vi "read data type.vi"(8 "error in":errorcluster, 11 "system tag in":refnum<class "tag descriptor.lvclass">) -> (0 "error out":errorcluster, 2 "data type":T1, 3 "system tag out":refnum<class "tag descriptor.lvclass">)   [LabVIEW 2013, in "tag bus.lvlib" / "tag descriptor.lvclass"]
doc: "Read the value of the data type enum in a given tag descriptor."
uses:
  tag descriptor.lvclass
  Data Type.ctl
  tag descriptor.lvclass/tag descriptor.ctl
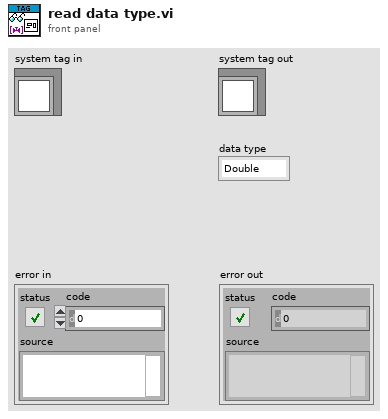
[diagram p1: front panel]
types:
  T1 = typedef "tag bus.lvlib/tag descriptor.lvclass/Data Type.ctl" = enum16{"Double", "Single", "I64", "I32", "I16", "I8", "U64", "U32", "U16", "U8", "Boolean", "String", "Array of Double", "Array of Single", "Array of I64", "Array of I32", "Array of I16", "Array of I8", "Array of U64", "Array of U32", "Array of U16", "Array of U8", "Array of Boolean", "Array of String"}
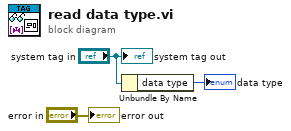
[diagram p0: block diagram]
diagram:
  n1 = Unbundle By Name("system tag in") -> ("data type"=→"data type":T1)
  "system tag out" <- "system tag in"
  "error out" <- "error in"
